vi "TIO RPC Notification U8.vi"(4 "Notification Prefix":string, 7 "error in (no error)":errorcluster, 8 "U8":u8, 9 "Read":bool, 10 "String":string) -> (0 "error out":errorcluster, 1 "U8":u8, 2 "Response":bool)   [LabVIEW 2017]
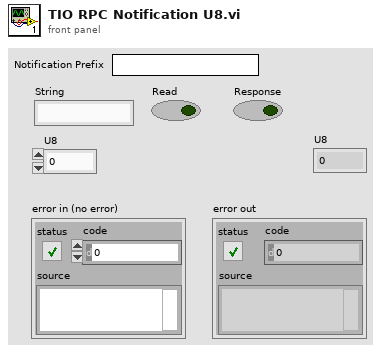
[diagram p1: front panel]
types:
  T1 = enum16{"big-endian, network order", "native, host order", "little-endian"}
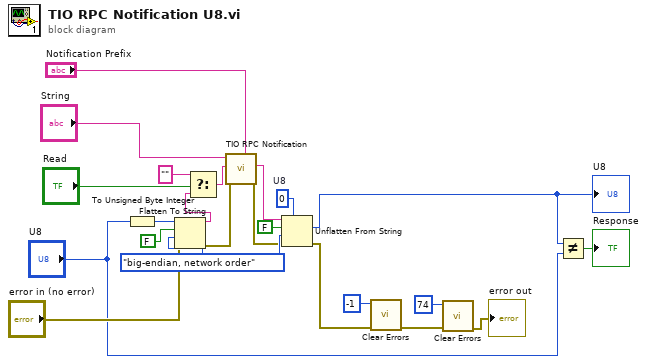
[diagram p0: block diagram]
diagram:
  w23 = u8 0  # U8
  w20 = T1."big-endian, network order" ("byte order (0:big-endian, network order)")
  n1 = To Unsigned Byte Integer(number="U8") -> (unsigned 8bit integer=w15:u8)
  n2 = Flatten To String(anything=w15, prepend array or string size? (T)=FALSE, byte order (0:big-endian, network order)=w20, error in (no error)="error in (no error)") -> (data string=w17:string, error out=w11:errorcluster)  [unwired: 1 out]
  n3 = Select(t="", s="Read", f=w17) -> (s? t:f=w16:string)
  n4 = call "TIO RPC Notification.vi"("Notification Prefix"="Notification Prefix", "error in (no error)"=w11, "Payload"=w16, "Topic"="String") -> ("error out"=w3:errorcluster, "REP"=w21:string)  [unwired: 4 in, 1 out]
  n5 = Unflatten From String(type=w23, binary string=w21, data includes array or string size? (T)=FALSE, byte order (0:big-endian, network order)=w20, error in (no error)=w3) -> (value=w1:u8, error out=w7:errorcluster)  [unwired: 1 out]
  "U8" <- w1
  n6 = call <vilib>:"Clear Errors.vi"("error in (no error)"=w7, "specific error code to clear (0: all)"=-1) -> ("error out"=w9:errorcluster)  [unwired: 4 in, 1 out]
  n7 = call <vilib>:"Clear Errors.vi"("error in (no error)"=w9, "specific error code to clear (0: all)"=74) -> ("error out"=→"error out":errorcluster)  [unwired: 4 in, 1 out]
  n8 = Not Equal?(x=w1, y="U8") -> (x != y?=→"Response":bool)
